vi "ex4-1.vi"   [LabVIEW 2009]
uses:
  <vilib>/NXT/Dual Mode Library/Display/drawNumber.vi
  <vilib>/NXT/Dual Mode Library/Waits/Wait_Num.vi
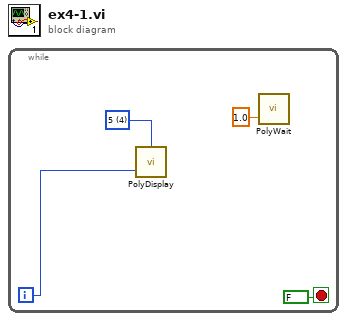
[diagram p0: block diagram]
diagram:
  n1 = while {
    i -> [w3]
    stop <- FALSE stop-if-true
    w2 = i16 4 items=["1", "2", "3", "4", "5", "6", "7", "8"] ("Line")
    n2 = call-poly <vilib>:"PolyDisplay.vi"("number"=w3, "Line"=w2) -> ()  [unwired: 2 in, 1 out]
    n3 = call-poly <vilib>:"PolyWait.vi"("Time (1 sec)"=sgl 1.0) -> ()  [unwired: 3 in, 1 out]
  }
